vi "List All Jobs.vi"(0 "SystemLink repo in":T2, 11 "error in (no error)":errorcluster) -> (4 "SystemLink repo out":T2, 6 "jobs":T1[](array[typedef]), 15 "error out":errorcluster)   [LabVIEW 2017, in "SystemLink_Repo_API.lvlib"]
doc: "Lists the data for all jobs.\nNote: Jobs are automtically deleted after they are 30 days old."
uses:
  SystemLink_Repo_API.lvlib
  <vilib>/httpClient/LabVIEWHTTPClient.lvlib
  syslink_jobs.ctl
  syslink_job_datatype.ctl
  <vilib>/httpClient/ClientHandle.ctl
  systemlink repo.ctl
panel:
  out "body":string
  out "headers":string
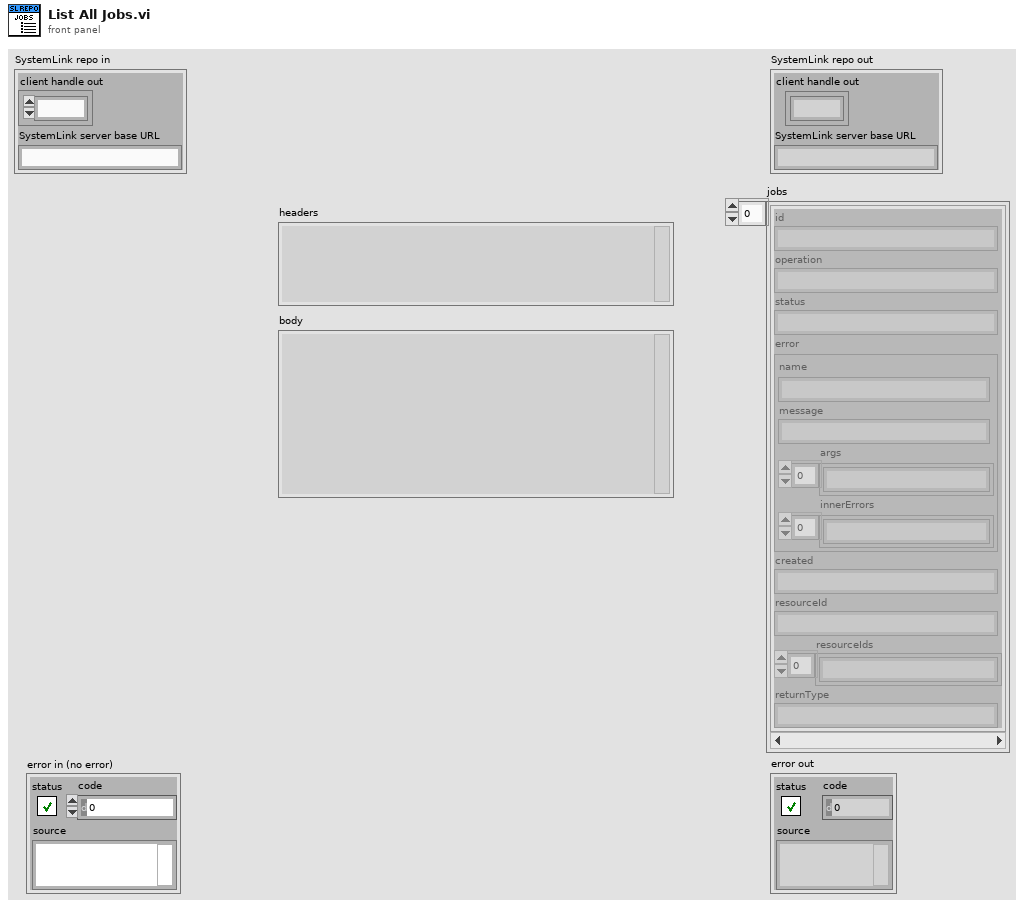
[diagram p1: front panel]
types:
  T1 = typedef "SystemLink_Repo_API.lvlib/syslink_job_datatype.ctl" = cluster{"id":string, "operation":string, "status":string, "error":cluster{"name":string, "message":string, "args":string[], "innerErrors":string[]}, "created":string, "resourceId":string, "resourceIds":string[], "returnType":string}
  T2 = typedef "SystemLink_Repo_API.lvlib/systemlink repo.ctl" = cluster{"client handle out":T3, "SystemLink server base URL":string}
  T3 = typedef "LabVIEWHTTPClient.lvlib/ClientHandle.ctl" = refnum<k1>
  T4 = typedef "SystemLink_Repo_API.lvlib/syslink_jobs.ctl" = cluster{"jobs":T1[]}
  T5 = cluster{"id":string, "operation":string, "status":string, "error":string[], "created":string, "resourceId":string, "resourceIds":string[], "returnType":string}[]
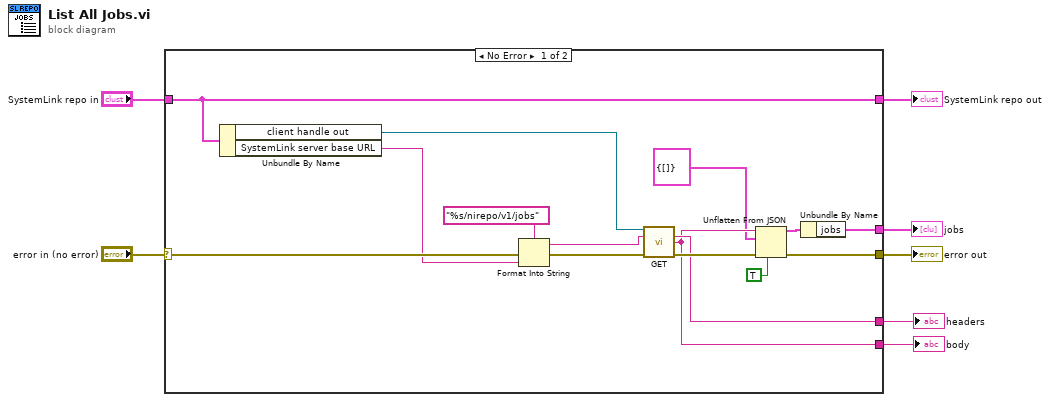
[diagram p0: block diagram]
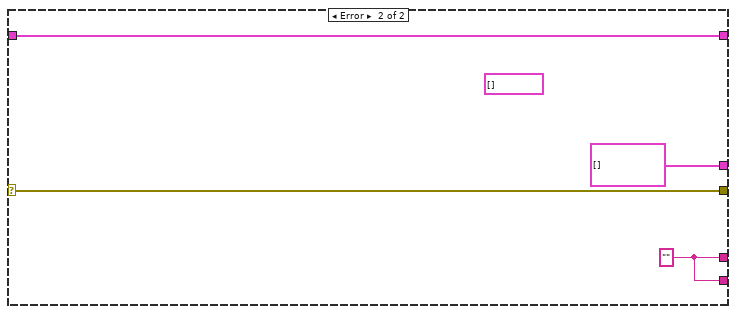
[diagram p2: hidden frame]
diagram:
  n1 = case shown="No Error" "error in (no error)" {
    selector: "error in (no error)" -> [w19 w26]
    tunnel: "SystemLink repo in" -> [w8 w23]
    tunnel: [w14 w26] -> w6
    tunnel: [w13 w25] -> w5
    tunnel: [w15 w25] -> w4
    tunnel: [w9 T1[] [] ("jobs")] -> w3
    tunnel: [w8 w23] -> w2
    frame No Error {
      n2 = Unbundle By Name(w8) -> ("client handle out"=w20:T3, "SystemLink server base URL"=w16:string)
      n3 = Format Into String(format string="%s/nirepo/v1/jobs", error in=w19, w16) -> (resulting string=w21:string, error out=w18:errorcluster)  [unwired: 1 in]
      n4 = call <vilib>:"GET.vi"("client handle"=w20, "url"=w21, "error in (no error)"=w18) -> ("headers"=w15:string, "body"=w13:string, "error out"=w17:errorcluster)  [unwired: 9 in, 1 out]
      n5 = Unflatten From JSON(JSON string=w13, type and defaults=T4 {"jobs"=[]} ("syslink_jobs"), default null elements? (F)=TRUE, error in (no error)=w17) -> (value=w10:T4, error out=w14:errorcluster)  [unwired: 3 in]
      n6 = Unbundle By Name(w10) -> ("jobs"=w9:T1[])
    }
    frame Error {
      (unwired) T5 [] ("jobs")
      w25 = "" ("headers")
    }
  }
  "error out" <- w6
  "SystemLink repo out" <- w2
  "headers" <- w4
  "body" <- w5
  "jobs" <- w3
